vi "read Log11 emibin record.vi"(0 "refnum in":refnum<file>, 7 "Log11 File Metrix":T1, 9 "Package(-1, Next)":i32=-1, 11 "error in":errorcluster) -> (4 "refnum out":refnum<file>, 6 "record time":timestamp, 8 "Doubles":dbl[](array[numeric]), 10 "U8 std":u8[](array[numeric]), 15 "error out":errorcluster)   [LabVIEW 2011]
uses:
  Log11 emibin file Metrix.ctl
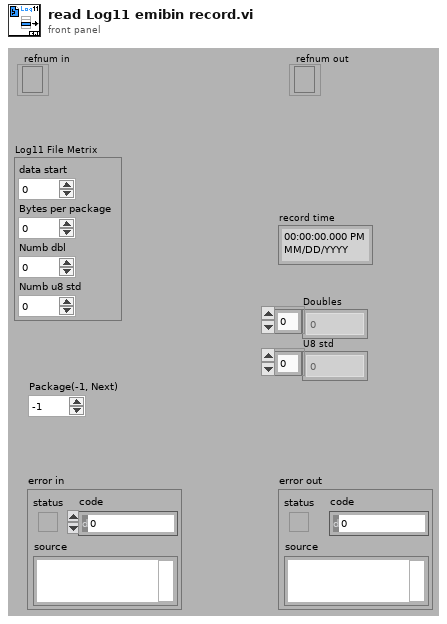
[diagram p1: front panel]
types:
  T1 = typedef "Log11 emibin file Metrix.ctl" = cluster{"data start":u32, "Bytes per package":i32, "Numb dbl":i32, "Numb u8 std":i32}
  T2 = enum16{"big-endian, network order", "native, host order", "little-endian"}
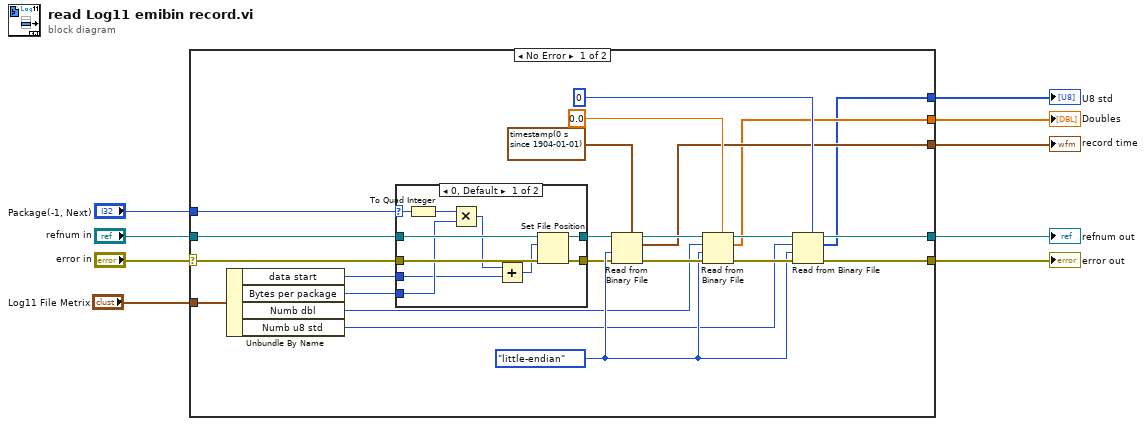
[diagram p0: block diagram]
diagram:
  n1 = case shown="No Error" "error in" {
    selector: "error in" -> [w13 w45]
    tunnel: [w29 w46] -> w9
    tunnel: [w26 w45] -> w8
    tunnel: "Log11 File Metrix" -> [w22 _]
    tunnel: "refnum in" -> [w17 w46]
    tunnel: "Package(-1, Next)" -> [w16 _]
    tunnel: [w12 _] -> w3
    tunnel: [w11 _] -> w2
    tunnel: [w10 _] -> w1
    frame No Error {
      w23 = T2."little-endian" ("byte order (0:big-endian, network order)")
      n2 = Unbundle By Name(w22) -> ("data start"=w15:u32, "Bytes per package"=w14:i32, "Numb dbl"=w21:i32, "Numb u8 std"=w20:i32)
      n3 = case shown="0, Default" w16 {
        selector: w16 -> [w38 _]
        tunnel: w13 -> [w42 w44]
        tunnel: [w41 w44] -> w19
        tunnel: [w40 w43] -> w18
        tunnel: w17 -> [w39 w43]
        tunnel: w15 -> [w36 _]
        tunnel: w14 -> [w37 _]
        frame 0, Default {
          n4 = To Quad Integer(1:w38) -> (0:w34:i64)
          n5 = Multiply(x=w34, y=w37) -> (x*y=w35:i64)
          n6 = Add(x=w35, y=w36) -> (x+y=w33:i64)
          n7 = Set File Position(offset (in bytes) (0)=w33, refnum=w39, error in=w42) -> (refnum out=w40:refnum<file>, error out=w41:errorcluster)  [unwired: 1 in]
        }
        frame -1 {
          # "Leser neste record"
        }
      }
      n8 = Read from Binary File(5:timestamp(0 s since 1904-01-01) ("current time"), 8:w19, 9:w23, 11:w18) -> (0:w24:errorcluster, 2:w12:timestamp, 3:w27:refnum<file>)  [unwired: 2 in, 1 out]
      n9 = Read from Binary File(5:0.0 ("number: 0 to 1"), 8:w24, 9:w23, 10:w21, 11:w27) -> (0:w25:errorcluster, 2:w11:dbl[], 3:w28:refnum<file>)  [unwired: 1 in, 1 out]
      n10 = Read from Binary File(5:u8 0, 8:w25, 9:w23, 10:w20, 11:w28) -> (0:w26:errorcluster, 2:w10:u8[], 3:w29:refnum<file>)  [unwired: 1 in, 1 out]
    }
    frame Error {
    }
  }
  "refnum out" <- w9
  "error out" <- w8
  "record time" <- w3
  "Doubles" <- w2
  "U8 std" <- w1
